vi "Lab Panel V4.85.vi"() -> ()   [LabVIEW 2013] (continued)
                            n1529 = local write "run lab03-2"(w2748) -> ()
                          }
                          frame #1 {
                            n1530 = TDMS Close(11:w2752) -> (0:w2753:errorcluster)  [unwired: 1 in, 1 out]
                            n1531 = local write "data file error"(w2753) -> ()
                          }
                          frame #2 {
                            n1532 = stacked-sequence {
                              tunnel: "LAB03-2" -> [w2761 w2762]
                              tunnel: w2758 -> [_ w2767]
                              tunnel: w2757 -> [_ w2766]
                              tunnel: w2756 -> [_ w2765]
                              tunnel: w2755 -> [_ w2764]
                              tunnel: w2754 -> [_ w2763]
                              frame #0 {
                                n1533 = call "sub vi - defrag tdms v1.vi"("panel id"=w2761) -> ("error out"=w2760:errorcluster)  [unwired: 10 in]
                                n1534 = local write "data file error"(w2760) -> ()
                              }
                              frame #1 {
                                n1535 = Bundle("STATUS"=w2767, "OUT SERVER ADDRESS"=w2766, "FROM ACCOUNT"=w2765, "Test File To"=w2764, "Mail Test Fail"=w2763) -> (w2769:T23)  [unwired: 1 in]
                                n1536 = call "Save data file to network drive v3.vi"("Input Cluster"=w2769, "panel id"=w2762) -> ("network file save error"=w2768:errorcluster)  [unwired: 8 in, 1 out]
                                n1537 = local write "data file error"(w2768) -> ()
                              }
                            }
                          }
                        }
                      }
                    }
                  }
                }
              }
              frame #6 {
                # "LAB04-1"
                n1538 = local read "run lab04-1"() -> (w2774:bool)
                n1539 = case shown="True" w2774 {
                  tunnel: w2773 -> [_ w2778]
                  tunnel: w2772 -> [_ w2777]
                  tunnel: w2771 -> [_ w2776]
                  tunnel: w2770 -> [_ w2775]
                  frame False {
                  }
                  frame True {
                    n1540 = local read "DISP LAB04-1"() -> (w2786:T4)
                    n1541 = Unbundle(w2786) -> ("CYCLE"=w2782:dbl, "STATUS"=w2779:string)  [unwired: 1 out]
                    n1542 = local read "TDMS LAB04-1"() -> (w2785:refnum<k34>)
                    n1543 = Not Equal?(x=w2779, y="RUN") -> (x != y?=w2781:bool)
                    n1544 = Greater?(x=w2782, y=2.0) -> (0:w2783:bool)
                    n1545 = And(x=w2783, y=w2781) -> (x .and. y?=w2780:bool)
                    n1546 = case shown="True" w2780 {
                      tunnel: w2786 -> [_ w2794]
                      tunnel: w2785 -> [_ w2793]
                      tunnel: w2779 -> [_ w2792]
                      tunnel: w2778 -> [_ w2791]
                      tunnel: w2777 -> [_ w2790]
                      tunnel: w2776 -> [_ w2789]
                      tunnel: w2775 -> [_ w2788]
                      frame False {
                      }
                      frame True {
                        n1547 = stacked-sequence {
                          tunnel: w2794 -> [w2797 _ _]
                          tunnel: w2793 -> [_ w2799 _]
                          tunnel: w2792 -> [_ _ w2805]
                          tunnel: w2791 -> [_ _ w2804]
                          tunnel: w2790 -> [_ _ w2803]
                          tunnel: w2789 -> [_ _ w2802]
                          tunnel: w2788 -> [_ _ w2801]
                          frame #0 {
                            w2795 = FALSE
                            n1548 = local write "mail control"("END") -> ()
                            n1549 = Bundle(cluster=w2797) -> (w2798:T4)  [unwired: 3 in]
                            n1550 = local write "RUN LAB04-1"(w2795) -> ()
                            n1551 = local write "O/I  LAB04-1"(w2795) -> ()
                            n1552 = local write "run lab04-1"(w2795) -> ()
                            n1553 = local write "DISP LAB04-1"(w2798) -> ()
                          }
                          frame #1 {
                            n1554 = TDMS Close(11:w2799) -> (0:w2800:errorcluster)  [unwired: 1 in, 1 out]
                            n1555 = local write "data file error"(w2800) -> ()
                          }
                          frame #2 {
                            n1556 = stacked-sequence {
                              tunnel: "LAB04-1" -> [w2808 w2809]
                              tunnel: w2805 -> [_ w2814]
                              tunnel: w2804 -> [_ w2813]
                              tunnel: w2803 -> [_ w2812]
                              tunnel: w2802 -> [_ w2811]
                              tunnel: w2801 -> [_ w2810]
                              frame #0 {
                                n1557 = call "sub vi - defrag tdms v1.vi"("panel id"=w2808) -> ("error out"=w2807:errorcluster)  [unwired: 10 in]
                                n1558 = local write "data file error"(w2807) -> ()
                              }
                              frame #1 {
                                n1559 = Bundle("STATUS"=w2814, "OUT SERVER ADDRESS"=w2813, "FROM ACCOUNT"=w2812, "Test File To"=w2811, "Mail Test Fail"=w2810) -> (w2816:T23)  [unwired: 1 in]
                                n1560 = call "Save data file to network drive v3.vi"("Input Cluster"=w2816, "panel id"=w2809) -> ("network file save error"=w2815:errorcluster)  [unwired: 8 in, 1 out]
                                n1561 = local write "data file error"(w2815) -> ()
                              }
                            }
                          }
                        }
                      }
                    }
                  }
                }
              }
              frame #7 {
                # "LAB04-2"
                n1562 = local read "run lab04-2"() -> (w2821:bool)
                n1563 = case shown="True" w2821 {
                  tunnel: w2820 -> [_ w2825]
                  tunnel: w2819 -> [_ w2824]
                  tunnel: w2818 -> [_ w2823]
                  tunnel: w2817 -> [_ w2822]
                  frame False {
                  }
                  frame True {
                    n1564 = local read "DISP LAB04-2"() -> (w2833:T4)
                    n1565 = Unbundle(w2833) -> ("CYCLE"=w2829:dbl, "STATUS"=w2826:string)  [unwired: 1 out]
                    n1566 = Not Equal?(x=w2826, y="RUN") -> (x != y?=w2828:bool)
                    n1567 = local read "TDMS LAB04-2"() -> (w2832:refnum<k34>)
                    n1568 = Greater?(x=w2829, y=2.0) -> (0:w2830:bool)
                    n1569 = And(x=w2830, y=w2828) -> (x .and. y?=w2827:bool)
                    n1570 = case shown="True" w2827 {
                      tunnel: w2833 -> [_ w2841]
                      tunnel: w2832 -> [_ w2840]
                      tunnel: w2826 -> [_ w2839]
                      tunnel: w2825 -> [_ w2838]
                      tunnel: w2824 -> [_ w2837]
                      tunnel: w2823 -> [_ w2836]
                      tunnel: w2822 -> [_ w2835]
                      frame False {
                      }
                      frame True {
                        n1571 = stacked-sequence {
                          tunnel: w2841 -> [w2844 _ _]
                          tunnel: w2840 -> [_ w2846 _]
                          tunnel: w2839 -> [_ _ w2852]
                          tunnel: w2838 -> [_ _ w2851]
                          tunnel: w2837 -> [_ _ w2850]
                          tunnel: w2836 -> [_ _ w2849]
                          tunnel: w2835 -> [_ _ w2848]
                          frame #0 {
                            w2842 = FALSE
                            n1572 = local write "mail control"("END") -> ()
                            n1573 = Bundle(cluster=w2844) -> (w2845:T4)  [unwired: 3 in]
                            n1574 = local write "O/I  LAB04-2"(w2842) -> ()
                            n1575 = local write "RUN LAB04-2"(w2842) -> ()
                            n1576 = local write "run lab04-2"(w2842) -> ()
                            n1577 = local write "DISP LAB04-2"(w2845) -> ()
                          }
                          frame #1 {
                            n1578 = TDMS Close(11:w2846) -> (0:w2847:errorcluster)  [unwired: 1 in, 1 out]
                            n1579 = local write "data file error"(w2847) -> ()
                          }
                          frame #2 {
                            n1580 = stacked-sequence {
                              tunnel: "LAB04-2" -> [w2855 w2856]
                              tunnel: w2852 -> [_ w2861]
                              tunnel: w2851 -> [_ w2860]
                              tunnel: w2850 -> [_ w2859]
                              tunnel: w2849 -> [_ w2858]
                              tunnel: w2848 -> [_ w2857]
                              frame #0 {
                                n1581 = call "sub vi - defrag tdms v1.vi"("panel id"=w2855) -> ("error out"=w2854:errorcluster)  [unwired: 10 in]
                                n1582 = local write "data file error"(w2854) -> ()
                              }
                              frame #1 {
                                n1583 = Bundle("STATUS"=w2861, "OUT SERVER ADDRESS"=w2860, "FROM ACCOUNT"=w2859, "Test File To"=w2858, "Mail Test Fail"=w2857) -> (w2863:T23)  [unwired: 1 in]
                                n1584 = call "Save data file to network drive v3.vi"("Input Cluster"=w2863, "panel id"=w2856) -> ("network file save error"=w2862:errorcluster)  [unwired: 8 in, 1 out]
                                n1585 = local write "data file error"(w2862) -> ()
                              }
                            }
                          }
                        }
                      }
                    }
                  }
                }
              }
              frame #8 {
                # "LAB05-1"
                n1586 = local read "run lab05-1"() -> (w2868:bool)
                n1587 = case shown="True" w2868 {
                  tunnel: w2867 -> [_ w2872]
                  tunnel: w2866 -> [_ w2871]
                  tunnel: w2865 -> [_ w2870]
                  tunnel: w2864 -> [_ w2869]
                  frame False {
                  }
                  frame True {
                    n1588 = local read "DISP LAB05-1"() -> (w2880:T4)
                    n1589 = Unbundle(w2880) -> ("CYCLE"=w2876:dbl, "STATUS"=w2873:string)  [unwired: 1 out]
                    n1590 = Not Equal?(x=w2873, y="RUN") -> (x != y?=w2875:bool)
                    n1591 = local read "TDMS LAB05-1"() -> (w2879:refnum<k34>)
                    n1592 = Greater?(x=w2876, y=2.0) -> (0:w2877:bool)
                    n1593 = And(x=w2877, y=w2875) -> (x .and. y?=w2874:bool)
                    n1594 = case shown="True" w2874 {
                      tunnel: w2880 -> [_ w2888]
                      tunnel: w2879 -> [_ w2887]
                      tunnel: w2873 -> [_ w2886]
                      tunnel: w2872 -> [_ w2885]
                      tunnel: w2871 -> [_ w2884]
                      tunnel: w2870 -> [_ w2883]
                      tunnel: w2869 -> [_ w2882]
                      frame False {
                      }
                      frame True {
                        n1595 = stacked-sequence {
                          tunnel: w2888 -> [w2891 _ _]
                          tunnel: w2887 -> [_ w2893 _]
                          tunnel: w2886 -> [_ _ w2899]
                          tunnel: w2885 -> [_ _ w2898]
                          tunnel: w2884 -> [_ _ w2897]
                          tunnel: w2883 -> [_ _ w2896]
                          tunnel: w2882 -> [_ _ w2895]
                          frame #0 {
                            w2889 = FALSE
                            n1596 = local write "mail control"("END") -> ()
                            n1597 = Bundle(cluster=w2891) -> (w2892:T4)  [unwired: 3 in]
                            n1598 = local write "O/I  LAB05-1"(w2889) -> ()
                            n1599 = local write "RUN LAB05-1"(w2889) -> ()
                            n1600 = local write "run lab05-1"(w2889) -> ()
                            n1601 = local write "DISP LAB05-1"(w2892) -> ()
                          }
                          frame #1 {
                            n1602 = TDMS Close(11:w2893) -> (0:w2894:errorcluster)  [unwired: 1 in, 1 out]
                            n1603 = local write "data file error"(w2894) -> ()
                          }
                          frame #2 {
                            n1604 = stacked-sequence {
                              tunnel: "LAB05-1" -> [w2902 w2908]
                              tunnel: w2899 -> [_ w2907]
                              tunnel: w2898 -> [_ w2906]
                              tunnel: w2897 -> [_ w2905]
                              tunnel: w2896 -> [_ w2904]
                              tunnel: w2895 -> [_ w2903]
                              frame #0 {
                                n1605 = call "sub vi - defrag tdms v1.vi"("panel id"=w2902) -> ("error out"=w2901:errorcluster)  [unwired: 10 in]
                                n1606 = local write "data file error"(w2901) -> ()
                              }
                              frame #1 {
                                n1607 = Bundle("STATUS"=w2907, "OUT SERVER ADDRESS"=w2906, "FROM ACCOUNT"=w2905, "Test File To"=w2904, "Mail Test Fail"=w2903) -> (w2910:T23)  [unwired: 1 in]
                                n1608 = call "Save data file to network drive v3.vi"("Input Cluster"=w2910, "panel id"=w2908) -> ("network file save error"=w2909:errorcluster)  [unwired: 8 in, 1 out]
                                n1609 = local write "data file error"(w2909) -> ()
                              }
                            }
                          }
                        }
                      }
                    }
                  }
                }
              }
              frame #9 {
                # "LAB05-2"
                n1610 = local read "run lab05-2"() -> (w2915:bool)
                n1611 = case shown="True" w2915 {
                  tunnel: w2914 -> [_ w2919]
                  tunnel: w2913 -> [_ w2918]
                  tunnel: w2912 -> [_ w2917]
                  tunnel: w2911 -> [_ w2916]
                  frame False {
                  }
                  frame True {
                    n1612 = local read "DISP LAB05-2"() -> (w2927:T4)
                    n1613 = Unbundle(w2927) -> ("CYCLE"=w2923:dbl, "STATUS"=w2920:string)  [unwired: 1 out]
                    n1614 = Not Equal?(x=w2920, y="RUN") -> (x != y?=w2922:bool)
                    n1615 = local read "TDMS LAB05-2"() -> (w2926:refnum<k34>)
                    n1616 = Greater?(x=w2923, y=2.0) -> (0:w2924:bool)
                    n1617 = And(x=w2924, y=w2922) -> (x .and. y?=w2921:bool)
                    n1618 = case shown="True" w2921 {
                      tunnel: w2927 -> [_ w2935]
                      tunnel: w2926 -> [_ w2934]
                      tunnel: w2920 -> [_ w2933]
                      tunnel: w2919 -> [_ w2932]
                      tunnel: w2918 -> [_ w2931]
                      tunnel: w2917 -> [_ w2930]
                      tunnel: w2916 -> [_ w2929]
                      frame False {
                      }
                      frame True {
                        n1619 = stacked-sequence {
                          tunnel: w2935 -> [w2938 _ _]
                          tunnel: w2934 -> [_ w2940 _]
                          tunnel: w2933 -> [_ _ w2946]
                          tunnel: w2932 -> [_ _ w2945]
                          tunnel: w2931 -> [_ _ w2944]
                          tunnel: w2930 -> [_ _ w2943]
                          tunnel: w2929 -> [_ _ w2942]
                          frame #0 {
                            w2936 = FALSE
                            n1620 = local write "mail control"("END") -> ()
                            n1621 = Bundle(cluster=w2938) -> (w2939:T4)  [unwired: 3 in]
                            n1622 = local write "RUN LAB05-2"(w2936) -> ()
                            n1623 = local write "O/I  LAB05-2"(w2936) -> ()
                            n1624 = local write "run lab05-2"(w2936) -> ()
                            n1625 = local write "DISP LAB05-2"(w2939) -> ()
                          }
                          frame #1 {
                            n1626 = TDMS Close(11:w2940) -> (0:w2941:errorcluster)  [unwired: 1 in, 1 out]
                            n1627 = local write "data file error"(w2941) -> ()
                          }
                          frame #2 {
                            n1628 = stacked-sequence {
                              tunnel: "LAB05-2" -> [w2949 w2955]
                              tunnel: w2946 -> [_ w2954]
                              tunnel: w2945 -> [_ w2953]
                              tunnel: w2944 -> [_ w2952]
                              tunnel: w2943 -> [_ w2951]
                              tunnel: w2942 -> [_ w2950]
                              frame #0 {
                                n1629 = call "sub vi - defrag tdms v1.vi"("panel id"=w2949) -> ("error out"=w2948:errorcluster)  [unwired: 10 in]
                                n1630 = local write "data file error"(w2948) -> ()
                              }
                              frame #1 {
                                n1631 = Bundle("STATUS"=w2954, "OUT SERVER ADDRESS"=w2953, "FROM ACCOUNT"=w2952, "Test File To"=w2951, "Mail Test Fail"=w2950) -> (w2957:T23)  [unwired: 1 in]
                                n1632 = call "Save data file to network drive v3.vi"("Input Cluster"=w2957, "panel id"=w2955) -> ("network file save error"=w2956:errorcluster)  [unwired: 8 in, 1 out]
                                n1633 = local write "data file error"(w2956) -> ()
                              }
                            }
                          }
                        }
                      }
                    }
                  }
                }
              }
            }
            n1634 = local read "Network Directory"() -> (w2471:path)
            n1635 = global write "Global 1.vi" "Network Drive"(w2471) -> ()
          }
          frame #7 {
            # "disable functions"
            n1636 = stacked-sequence {
              tunnel: w2967 -> [w2981 _ w3038]
              tunnel: w2966 -> [w2976 _ w3037]
              tunnel: w2965 -> [w2975 _ w3036]
              tunnel: w2964 -> [w2973 _ w3035]
              tunnel: w2963 -> [w2974 _ w3034]
              tunnel: w2962 -> [_ w2998 w3033]
              tunnel: w2961 -> [_ w2999 w3032]
              tunnel: w2960 -> [_ w3000 w3031]
              tunnel: w2959 -> [_ w3001 w3030]
              tunnel: w2958 -> [_ w3002 w3029]
              frame #0 {
                n1637 = Select(t=2, s=w2973, f=0) -> (s? t:f=w2969:i32)
                n1638 = Select(t=2, s=w2975, f=0) -> (s? t:f=w2970:i32)
                n1639 = Select(t=2, s=w2974, f=0) -> (s? t:f=w2968:i32)
                n1640 = Select(t=2, s=w2981, f=0) -> (s? t:f=w2972:i32)
                n1641 = Select(t=2, s=w2976, f=0) -> (s? t:f=w2971:i32)
                n1642 = property on="SELECT LAB02-2" class="RadioBtnsControl (strict)"("DisabledEnum"=w2969) -> ()  [unwired: 2 in, 2 out]
                n1643 = property on="SELECT LAB02-1" class="RadioBtnsControl (strict)"("DisabledEnum"=w2970) -> ()  [unwired: 2 in, 2 out]
                n1644 = property on="SELECT LAB03-1" class="RadioBtnsControl (strict)"("DisabledEnum"=w2968) -> ()  [unwired: 2 in, 2 out]
                n1645 = property on="SELECT LAB01-1" class="RadioBtnsControl (strict)"("DisabledEnum"=w2972) -> ()  [unwired: 2 in, 2 out]
                n1646 = property on="SELECT LAB01-2" class="RadioBtnsControl (strict)"("DisabledEnum"=w2971) -> ()  [unwired: 2 in, 2 out]
                n1647 = Not(x=w2981) -> (.not. x?=w2982:bool)
                n1648 = property on="RESULT LAB01-1" class="Bool (strict)"("Visible"=w2982) -> ()  [unwired: 2 in, 2 out]
                n1649 = Not(x=w2976) -> (.not. x?=w2980:bool)
                n1650 = Not(x=w2975) -> (.not. x?=w2979:bool)
                n1651 = Not(x=w2973) -> (.not. x?=w2978:bool)
                n1652 = property on="RESULT LAB01-2" class="Bool (strict)"("Visible"=w2980) -> ()  [unwired: 2 in, 2 out]
                n1653 = Not(x=w2974) -> (.not. x?=w2977:bool)
                n1654 = property on="RESULT LAB02-1" class="Bool (strict)"("Visible"=w2979) -> ()  [unwired: 2 in, 2 out]
                n1655 = property on="RESULT LAB02-2" class="Bool (strict)"("Visible"=w2978) -> ()  [unwired: 2 in, 2 out]
                n1656 = property on="RESULT LAB03-1" class="Bool (strict)"("Visible"=w2977) -> ()  [unwired: 2 in, 2 out]
                n1657 = property on="SET LAB01-1" class="Clust (strict)"("DisabledEnum"=w2972) -> ()  [unwired: 2 in, 2 out]
                n1658 = property on="SET LAB01-2" class="Clust (strict)"("DisabledEnum"=w2971) -> ()  [unwired: 2 in, 2 out]
                n1659 = property on="SET LAB02-1" class="Clust (strict)"("DisabledEnum"=w2970) -> ()  [unwired: 2 in, 2 out]
                n1660 = property on="SET LAB02-2" class="Clust (strict)"("DisabledEnum"=w2969) -> ()  [unwired: 2 in, 2 out]
                n1661 = property on="SET LAB03-1" class="Clust (strict)"("DisabledEnum"=w2968) -> ()  [unwired: 2 in, 2 out]
                n1662 = property on="O/I  LAB01-1" class="Bool (strict)"("DisabledEnum"=w2972) -> ()  [unwired: 2 in, 2 out]
                n1663 = property on="O/I  LAB01-2" class="Bool (strict)"("DisabledEnum"=w2971) -> ()  [unwired: 2 in, 2 out]
                n1664 = property on="O/I  LAB02-1" class="Bool (strict)"("DisabledEnum"=w2970) -> ()  [unwired: 2 in, 2 out]
                n1665 = property on="O/I  LAB02-2" class="Bool (strict)"("DisabledEnum"=w2969) -> ()  [unwired: 2 in, 2 out]
                n1666 = property on="O/I  LAB03-1" class="Bool (strict)"("DisabledEnum"=w2968) -> ()  [unwired: 2 in, 2 out]
              }
              frame #1 {
                n1667 = Select(t=2, s=w3002, f=0) -> (s? t:f=w2993:i32)
                n1668 = Select(t=2, s=w3001, f=0) -> (s? t:f=w2994:i32)
                n1669 = Select(t=2, s=w2998, f=0) -> (s? t:f=w2997:i32)
                n1670 = Select(t=2, s=w2999, f=0) -> (s? t:f=w2996:i32)
                n1671 = Select(t=2, s=w3000, f=0) -> (s? t:f=w2995:i32)
                n1672 = property on="SELECT LAB05-2" class="RadioBtnsControl (strict)"("DisabledEnum"=w2993) -> ()  [unwired: 2 in, 2 out]
                n1673 = property on="SELECT LAB05-1" class="RadioBtnsControl (strict)"("DisabledEnum"=w2994) -> ()  [unwired: 2 in, 2 out]
                n1674 = property on="SELECT LAB03-2" class="RadioBtnsControl (strict)"("DisabledEnum"=w2997) -> ()  [unwired: 2 in, 2 out]
                n1675 = property on="SELECT LAB04-1" class="RadioBtnsControl (strict)"("DisabledEnum"=w2996) -> ()  [unwired: 2 in, 2 out]
                n1676 = property on="SELECT LAB04-2" class="RadioBtnsControl (strict)"("DisabledEnum"=w2995) -> ()  [unwired: 2 in, 2 out]
                n1677 = property on="SET LAB05-2" class="Clust (strict)"("DisabledEnum"=w2993) -> ()  [unwired: 2 in, 2 out]
                n1678 = property on="SET LAB05-1" class="Clust (strict)"("DisabledEnum"=w2994) -> ()  [unwired: 2 in, 2 out]
                n1679 = property on="SET LAB03-2" class="Clust (strict)"("DisabledEnum"=w2997) -> ()  [unwired: 2 in, 2 out]
                n1680 = property on="SET LAB04-1" class="Clust (strict)"("DisabledEnum"=w2996) -> ()  [unwired: 2 in, 2 out]
                n1681 = property on="SET LAB04-2" class="Clust (strict)"("DisabledEnum"=w2995) -> ()  [unwired: 2 in, 2 out]
                n1682 = property on="O/I  LAB05-2" class="Bool (strict)"("DisabledEnum"=w2993) -> ()  [unwired: 2 in, 2 out]
                n1683 = property on="O/I  LAB05-1" class="Bool (strict)"("DisabledEnum"=w2994) -> ()  [unwired: 2 in, 2 out]
                n1684 = property on="O/I  LAB04-1" class="Bool (strict)"("DisabledEnum"=w2996) -> ()  [unwired: 2 in, 2 out]
                n1685 = property on="O/I  LAB04-2" class="Bool (strict)"("DisabledEnum"=w2995) -> ()  [unwired: 2 in, 2 out]
                n1686 = property on="O/I  LAB03-2" class="Bool (strict)"("DisabledEnum"=w2997) -> ()  [unwired: 2 in, 2 out]
                n1687 = Not(x=w3002) -> (.not. x?=w3003:bool)
                n1688 = Not(x=w3001) -> (.not. x?=w3004:bool)
                n1689 = Not(x=w3000) -> (.not. x?=w3005:bool)
                n1690 = property on="RESULT LAB05-2" class="Bool (strict)"("Visible"=w3003) -> ()  [unwired: 2 in, 2 out]
                n1691 = property on="RESULT LAB05-1" class="Bool (strict)"("Visible"=w3004) -> ()  [unwired: 2 in, 2 out]
                n1692 = Not(x=w2999) -> (.not. x?=w3006:bool)
                n1693 = property on="RESULT LAB04-2" class="Bool (strict)"("Visible"=w3005) -> ()  [unwired: 2 in, 2 out]
                n1694 = Not(x=w2998) -> (.not. x?=w3007:bool)
                n1695 = property on="RESULT LAB04-1" class="Bool (strict)"("Visible"=w3006) -> ()  [unwired: 2 in, 2 out]
                n1696 = property on="RESULT LAB03-2" class="Bool (strict)"("Visible"=w3007) -> ()  [unwired: 2 in, 2 out]
              }
              frame #2 {
                # "disable calibrate if any test running"
                n1697 = Or(x=w3030, y=w3029) -> (x .or. y?=w3023:bool)
                n1698 = Or(x=w3032, y=w3031) -> (x .or. y?=w3025:bool)
                n1699 = Or(x=w3036, y=w3035) -> (x .or. y?=w3027:bool)
                n1700 = Or(x=w3034, y=w3033) -> (x .or. y?=w3026:bool)
                n1701 = Or(x=w3038, y=w3037) -> (x .or. y?=w3028:bool)
                n1702 = Or(x=w3026, y=w3025) -> (x .or. y?=w3024:bool)
                n1703 = Or(x=w3028, y=w3027) -> (x .or. y?=w3022:bool)
                n1704 = Or(x=w3024, y=w3023) -> (x .or. y?=w3021:bool)
                n1705 = Or(x=w3022, y=w3021) -> (x .or. y?=w3020:bool)
                n1706 = case shown="False" w3020 {
                  tunnel: [0 2] -> w3019
                  frame False {
                  }
                  frame True {
                  }
                }
                n1707 = property on="JIG TEST" class="Clust (strict)"("DisabledEnum"=w3019) -> ()  [unwired: 2 in, 2 out]
                n1708 = property on="Network Directory" class="Path"("DisabledEnum"=w3019) -> ()  [unwired: 2 in, 2 out]
                n1709 = property on="MAIL SETTINGS" class="Clust (strict)"("DisabledEnum"=w3019) -> ()  [unwired: 2 in, 2 out]
                n1710 = property on="SET (cal)" class="Bool (strict)"("DisabledEnum"=w3019) -> ()  [unwired: 2 in, 2 out]
                n1711 = property on="ADMIN" class="Bool (strict)"("DisabledEnum"=0) -> ()  [unwired: 2 in, 2 out]
              }
            }
          }
          frame #8 {
            # "drive jigs"
            n1712 = stacked-sequence {
              frame #0 {
                # "jig on"
                n1713 = local read "jig cycle"() -> (w3046:dbl)
                n1714 = property on="JIG TEST" class="Clust (strict)"() -> ("DisabledEnum"=w3043:T14)  [unwired: 2 in, 2 out]
                n1715 = Equal?(x=w3043, y=2) -> (x = y?=w3042:bool)
                n1716 = Equal?(x=w3046, y=0) -> (x = y?=w3044:bool)
                n1717 = And(x=w3044, y=w3042) -> (x .and. y?=w3041:bool)
                n1718 = case shown="True" w3041 {
                  frame False {
                  }
                  frame True {
                    n1719 = local read "run lab01-1"() -> (w3057:bool)
                    n1720 = local read "run lab01-2"() -> (w3056:bool)
                    n1721 = local read "run lab02-1"() -> (w3055:bool)
                    n1722 = local read "run lab02-2"() -> (w3054:bool)
                    n1723 = local read "run lab03-1"() -> (w3053:bool)
                    n1724 = local read "run lab03-2"() -> (w3052:bool)
                    n1725 = local read "run lab04-1"() -> (w3051:bool)
                    n1726 = local read "run lab04-2"() -> (w3050:bool)
                    n1727 = local read "run lab05-1"() -> (w3049:bool)
                    n1728 = local read "run lab05-2"() -> (w3048:bool)
                    n1729 = local write "JIG LAB03-2"(w3052) -> ()
                    n1730 = local write "JIG LAB01-1"(w3057) -> ()
                    n1731 = local write "JIG LAB01-2"(w3056) -> ()
                    n1732 = local write "JIG LAB02-1"(w3055) -> ()
                    n1733 = local write "JIG LAB02-2"(w3054) -> ()
                    n1734 = local write "JIG LAB03-1"(w3053) -> ()
                    n1735 = local write "JIG LAB04-1"(w3051) -> ()
                    n1736 = local write "JIG LAB04-2"(w3050) -> ()
                    n1737 = local write "JIG LAB05-1"(w3049) -> ()
                    n1738 = local write "JIG LAB05-2"(w3048) -> ()
                  }
                }
              }
              frame #1 {
                # "jig off"
                n1739 = local read "jig cycle"() -> (w3064:dbl)
                n1740 = local read "on loops"() -> (w3063:dbl)
                n1741 = property on="JIG TEST" class="Clust (strict)"() -> ("DisabledEnum"=w3062:T14)  [unwired: 2 in, 2 out]
                n1742 = Equal?(x=w3062, y=2) -> (x = y?=w3060:bool)
                n1743 = Equal?(x=w3064, y=w3063) -> (x = y?=w3059:bool)
                n1744 = And(x=w3059, y=w3060) -> (x .and. y?=w3058:bool)
                n1745 = case shown="True" w3058 {
                  frame False {
                  }
                  frame True {
                    w3115 = FALSE
                    w3116 = TRUE
                    w3114 = 2
                    n1746 = local read "SELECT LAB05-2"() -> (w3105:T3)
                    n1747 = local read "SELECT LAB04-2"() -> (w3107:T3)
                    n1748 = local read "SELECT LAB04-1"() -> (w3108:T3)
                    n1749 = local read "SELECT LAB05-1"() -> (w3106:T3)
                    n1750 = local read "SELECT LAB03-2"() -> (w3109:T3)
                    n1751 = local read "SELECT LAB02-1"() -> (w3112:T3)
                    n1752 = local read "SELECT LAB03-1"() -> (w3110:T3)
                    n1753 = local read "SELECT LAB02-2"() -> (w3111:T3)
                    n1754 = local read "SELECT LAB01-2"() -> (w3113:T3)
                    n1755 = local read "run lab05-1"() -> (w3075:bool)
                    n1756 = local read "run lab05-2"() -> (w3074:bool)
                    n1757 = local read "SELECT LAB01-1"() -> (w3117:T3)
                    n1758 = local read "run lab04-2"() -> (w3076:bool)
                    n1759 = local read "run lab04-1"() -> (w3077:bool)
                    n1760 = local read "run lab01-1"() -> (w3093:bool)
                    n1761 = local read "run lab01-2"() -> (w3082:bool)
                    n1762 = local read "run lab03-2"() -> (w3078:bool)
                    n1763 = local read "run lab03-1"() -> (w3079:bool)
                    n1764 = local read "run lab02-1"() -> (w3081:bool)
                    n1765 = local read "run lab02-2"() -> (w3080:bool)
                    n1766 = Equal?(x=w3114, y=w3110) -> (x = y?=w3088:bool)
                    n1767 = Equal?(x=w3114, y=w3109) -> (x = y?=w3087:bool)
                    n1768 = Equal?(x=w3114, y=w3108) -> (x = y?=w3086:bool)
                    n1769 = Equal?(x=w3114, y=w3107) -> (x = y?=w3085:bool)
                    n1770 = Equal?(x=w3114, y=w3106) -> (x = y?=w3084:bool)
                    n1771 = Equal?(x=w3114, y=w3105) -> (x = y?=w3083:bool)
                    n1772 = Equal?(x=w3114, y=w3117) -> (x = y?=w3094:bool)
                    n1773 = Equal?(x=w3114, y=w3112) -> (x = y?=w3090:bool)
                    n1774 = Equal?(x=w3114, y=w3111) -> (x = y?=w3089:bool)
                    n1775 = Equal?(x=w3114, y=w3113) -> (x = y?=w3091:bool)
                    n1776 = And(x=w3085, y=w3076) -> (x .and. y?=w3067:bool)
                    n1777 = And(x=w3088, y=w3079) -> (x .and. y?=w3070:bool)
                    n1778 = And(x=w3086, y=w3077) -> (x .and. y?=w3068:bool)
                    n1779 = And(x=w3083, y=w3074) -> (x .and. y?=w3065:bool)
                    n1780 = And(x=w3089, y=w3080) -> (x .and. y?=w3071:bool)
                    n1781 = And(x=w3087, y=w3078) -> (x .and. y?=w3069:bool)
                    n1782 = And(x=w3084, y=w3075) -> (x .and. y?=w3066:bool)
                    n1783 = And(x=w3091, y=w3082) -> (x .and. y?=w3073:bool)
                    n1784 = And(x=w3094, y=w3093) -> (x .and. y?=w3092:bool)
                    n1785 = And(x=w3090, y=w3081) -> (x .and. y?=w3072:bool)
                    n1786 = Select(t=w3116, s=w3092, f=w3115) -> (s? t:f=w3095:bool)
                    n1787 = Select(t=w3116, s=w3073, f=w3115) -> (s? t:f=w3096:bool)
                    n1788 = Select(t=w3116, s=w3072, f=w3115) -> (s? t:f=w3097:bool)
                    n1789 = Select(t=w3116, s=w3071, f=w3115) -> (s? t:f=w3098:bool)
                    n1790 = Select(t=w3116, s=w3070, f=w3115) -> (s? t:f=w3099:bool)
                    n1791 = Select(t=w3116, s=w3069, f=w3115) -> (s? t:f=w3100:bool)
                    n1792 = Select(t=w3116, s=w3068, f=w3115) -> (s? t:f=w3101:bool)
                    n1793 = Select(t=w3116, s=w3067, f=w3115) -> (s? t:f=w3102:bool)
                    n1794 = Select(t=w3116, s=w3066, f=w3115) -> (s? t:f=w3103:bool)
                    n1795 = Select(t=w3116, s=w3065, f=w3115) -> (s? t:f=w3104:bool)
                    n1796 = local write "JIG LAB03-2"(w3100) -> ()
                    n1797 = local write "JIG LAB02-1"(w3097) -> ()
                    n1798 = local write "JIG LAB02-2"(w3098) -> ()
                    n1799 = local write "JIG LAB01-2"(w3096) -> ()
                    n1800 = local write "JIG LAB03-1"(w3099) -> ()
                    n1801 = local write "JIG LAB01-1"(w3095) -> ()
                    n1802 = local write "JIG LAB05-2"(w3104) -> ()
                    n1803 = local write "JIG LAB04-1"(w3101) -> ()
                    n1804 = local write "JIG LAB05-1"(w3103) -> ()
                    n1805 = local write "JIG LAB04-2"(w3102) -> ()
                  }
                }
              }
            }
          }
          frame #9 {
            # "enable  jig test output if no test busy"
            n1806 = property on="JIG TEST" class="Clust (strict)"() -> ("DisabledEnum"=w3120:T14)  [unwired: 2 in, 2 out]
            n1807 = Equal?(x=w3120, y=0) -> (x = y?=w3118:bool)
            n1808 = case shown="True" w3118 {
              frame False {
              }
              frame True {
                n1809 = local read "JIG TEST"() -> (w3131:T9)
                n1810 = Unbundle(w3131) -> ("LAB01-1"=w3130:bool, "LAB01-2"=w3129:bool, "LAB02-1"=w3128:bool, "LAB02-2"=w3127:bool, "LAB03-1"=w3126:bool, "LAB03-2"=w3125:bool, "LAB04-1"=w3124:bool, "LAB04-2"=w3123:bool, "LAB05-1"=w3122:bool, "LAB05-2"=w3121:bool)
                n1811 = local write "JIG LAB05-1"(w3122) -> ()
                n1812 = local write "JIG LAB05-2"(w3121) -> ()
                n1813 = local write "JIG LAB04-1"(w3124) -> ()
                n1814 = local write "JIG LAB04-2"(w3123) -> ()
                n1815 = local write "JIG LAB03-2"(w3125) -> ()
                n1816 = local write "JIG LAB01-1"(w3130) -> ()
                n1817 = local write "JIG LAB02-1"(w3128) -> ()
                n1818 = local write "JIG LAB03-1"(w3126) -> ()
                n1819 = local write "JIG LAB01-2"(w3129) -> ()
                n1820 = local write "JIG LAB02-2"(w3127) -> ()
              }
            }
          }
          frame #10 {
            # "drive digital output"
            n1821 = local read "O/I  LAB05-2"() -> (w3138:bool)
            n1822 = local read "O/I  LAB05-1"() -> (w3140:bool)
            n1823 = local read "JIG LAB05-2"() -> (w3137:bool)
            n1824 = local read "O/I  LAB04-2"() -> (w3142:bool)
            n1825 = local read "JIG LAB05-1"() -> (w3139:bool)
            n1826 = local read "JIG LAB04-2"() -> (w3141:bool)
            n1827 = local read "O/I  LAB03-1"() -> (w3147:bool)
            n1828 = local read "O/I  LAB04-1"() -> (w3143:bool)
            n1829 = local read "O/I  LAB02-1"() -> (w3151:bool)
            n1830 = local read "O/I  LAB02-2"() -> (w3149:bool)
            n1831 = local read "O/I  LAB03-2"() -> (w3145:bool)
            n1832 = local read "JIG LAB04-1"() -> (w3136:bool)
            n1833 = local read "JIG LAB03-2"() -> (w3144:bool)
            n1834 = local read "O/I  LAB01-2"() -> (w3153:bool)
            n1835 = local read "JIG LAB02-1"() -> (w3150:bool)
            n1836 = local read "JIG LAB02-2"() -> (w3148:bool)
            n1837 = local read "JIG LAB03-1"() -> (w3146:bool)
            n1838 = local read "O/I  LAB01-1"() -> (w3155:bool)
            n1839 = local read "JIG LAB01-2"() -> (w3152:bool)
            n1840 = local read "JIG LAB01-1"() -> (w3154:bool)
            n1841 = Build Array(w3142, w3141, w3140, w3139, w3138, w3137) -> (w3133:bool[])
            n1842 = Build Array(w3148, w3147, w3146, w3145, w3144, w3143, w3136) -> (w3134:bool[])
            n1843 = Build Array(w3155, w3154, w3153, w3152, w3151, w3150, w3149) -> (w3135:bool[])
            n1844 = local read "simulate"() -> (w3132:bool)
            n1845 = case shown="False" w3132 {
              tunnel: w3135 -> [w3158 _]
              tunnel: w3134 -> [w3157 _]
              tunnel: w3133 -> [w3156 _]
              frame False {
                n1846 = call "sub vi - Drive Relays All v6.vi"("Array #2"=w3156, "Array #1"=w3157, "Array #0"=w3158) -> ()  [unwired: 8 in, 1 out]
              }
              frame True {
              }
            }
          }
          frame #11 {
            # "get analog values"
            n1847 = local read "on loops"() -> (w3165:dbl)
            n1848 = local read "jig cycle"() -> (w3162:dbl)
            n1849 = Add(x=w3165, y=1) -> (x+y=w3163:dbl)
            n1850 = Equal?(x=w3162, y=1) -> (x = y?=w3160:bool)
            n1851 = Equal?(x=w3162, y=w3163) -> (x = y?=w3161:bool)
            n1852 = Or(x=w3160, y=w3161) -> (x .or. y?=w3159:bool)
            n1853 = case shown="True" w3159 {
              frame False {
              }
              frame True {
                n1854 = local read "simulate"() -> (w3169:bool)
                n1855 = case shown="False" w3169 {
                  tunnel: [w3185 errorcluster[] [] ("array ERROR")] -> w3177
                  tunnel: [w3184 0.3 ("Analog loop time")] -> w3176
                  tunnel: [w3183 dynamicdata[] [] ("array GRAPH")] -> w3175
                  tunnel: [w3182 w3187] -> w3174
                  tunnel: [w3181 w3187] -> w3173
                  tunnel: [w3180 w3187] -> w3172
                  tunnel: [w3179 w3187] -> w3171
                  tunnel: [w3178 w3187] -> w3170
                  frame False {
                    n1856 = call "sub vi - Read Analog All v8.vi"() -> ("Analog loop time"=w3184:dbl, "array GRAPH"=w3183:dynamicdata[], "LAB01"=w3182:T24, "LAB02"=w3181:T25, "LAB03"=w3180:T26, "LAB04"=w3179:T27, "array ERROR"=w3185:errorcluster[], "LAB05"=w3178:T28)  [unwired: 8 in]
                  }
                  frame True {
                    w3187 = T28 {"LAB05-1 (A)"=10.0, "LAB05-1 (V)"=220.0, "LAB05-1 (PF)"=0.5, "LAB05-2 (A)"=15.0, "LAB05-2 (V)"=225.0, "LAB05-2 (PF)"=0.6} ("LAB05")
                  }
                }
                n1857 = local read "simulate"() -> (w3168:bool)
                n1858 = stacked-sequence {
                  tunnel: w3177 -> [w3194 _ _ _ _ _]
                  tunnel: w3176 -> [w3193 _ _ _ _ _]
                  tunnel: w3175 -> [w3192 _ _ _ _ _]
                  tunnel: w3174 -> [_ w3241 _ _ _ _]
                  tunnel: w3173 -> [_ _ w3248 _ _ _]
                  tunnel: w3172 -> [_ _ _ w3277 _ _]
                  tunnel: w3171 -> [_ _ _ _ w3304 _]
                  tunnel: w3170 -> [_ _ _ _ _ w3333]
                  tunnel: w3168 -> [_ w3219 w3247 w3275 w3303 w3331]
                  tunnel: T12 {"1  (A) cal"=1.0, "1 (V) cal"=1.0, "1 (PF) cal"=1.0, "1 (TL) cal"=1.0, "1 (TN) cal"=1.0, "2 (A) cal"=1.0, "2 (V) cal"=1.0, "2 (PF) cal"=1.0, "2 (TL) cal"=1.0, "2 (TN) cal"=1.0} ("CAL LAB01") -> [_ w3218 w3246 w3274 w3302 w3330]
                  frame #0 {
                    n1859 = local write "AI"(TRUE) -> ()
                    n1860 = global write "Global 1.vi" "RATE(Hz)"("RATE (Hz)") -> ()
                    n1861 = global write "Global 1.vi" "SAMPLES"("SAMPLES") -> ()
                    n1862 = Index Array(array=w3192, index=6) -> (element=→"LAB04-1 (GRAPH)":dynamicdata)
                    n1863 = Index Array(array=w3192, index=7) -> (element=→"LAB04-2 (GRAPH)":dynamicdata)
                    n1864 = Index Array(array=w3192, index=9) -> (element=→"LAB05-2 (GRAPH)":dynamicdata)
                    n1865 = Index Array(array=w3192, index=8) -> (element=→"LAB05-1 (GRAPH)":dynamicdata)
                    n1866 = Index Array(array=w3192, index=5) -> (element=→"LAB03-2 (GRAPH)":dynamicdata)
                    n1867 = Index Array(array=w3192, index=0) -> (element=→"LAB01-1 (GRAPH)":dynamicdata)
                    n1868 = Index Array(array=w3192, index=1) -> (element=→"LAB01-2 (GRAPH)":dynamicdata)
                    n1869 = Index Array(array=w3192, index=2) -> (element=→"LAB02-1 (GRAPH)":dynamicdata)
                    n1870 = Index Array(array=w3192, index=3) -> (element=→"LAB02-2 (GRAPH)":dynamicdata)
                    n1871 = Index Array(array=w3192, index=4) -> (element=→"LAB03-1 (GRAPH)":dynamicdata)
                    "AI loop time" <- w3193
                    "Analog Error Array" <- w3194
                  }
                  frame #1 {
                    n1872 = Unbundle By Name(w3241) -> ("LAB05-1 (A)"=w3239:dbl, "LAB05-1 (V)"=w3238:dbl, "LAB05-1 (PF)"=w3237:dbl, "LAB05-2 (A)"=w3236:dbl, "LAB05-2 (V)"=w3235:dbl, "LAB05-2 (PF)"=w3234:dbl)
                    n1873 = case shown="False" w3219 {
                      tunnel: [w3242 w3243] -> w3240
                      tunnel: w3218 -> [_ w3243]
                      frame False {
                        n1874 = local read "CAL LAB01"() -> (w3242:T12)
                      }
                      frame True {
                      }
                    }
                    n1875 = Unbundle By Name(w3240) -> ("1  (A) cal"=w3233:dbl, "1 (V) cal"=w3232:dbl, "1 (PF) cal"=w3231:dbl, "2 (A) cal"=w3230:dbl, "2 (V) cal"=w3229:dbl, "2 (PF) cal"=w3228:dbl)  [unwired: 4 out]
                    n1876 = Multiply(x=w3239, y=w3233) -> (x*y=w3226:dbl)
                    n1877 = Multiply(x=w3238, y=w3232) -> (x*y=w3225:dbl)
                    n1878 = Multiply(x=w3237, y=w3231) -> (x*y=w3224:dbl)
                    n1879 = Multiply(x=w3236, y=w3230) -> (x*y=w3222:dbl)
                    n1880 = Multiply(x=w3235, y=w3229) -> (x*y=w3221:dbl)
                    n1881 = Multiply(x=w3234, y=w3228) -> (x*y=w3220:dbl)
                    n1882 = local read "SIG LAB01-1"() -> (w3227:T2)
                    n1883 = local read "SIG LAB01-2"() -> (w3223:T2)
                    n1884 = Bundle By Name(cluster=w3227, "AMPS"=w3226, "VOLTS"=w3225, "PF"=w3224) -> (w3217:T2)
                    n1885 = Bundle By Name(cluster=w3223, "AMPS"=w3222, "VOLTS"=w3221, "PF"=w3220) -> (w3216:T2)
                    n1886 = global write "Global display 1.vi" "SIG LAB01-2"(w3216) -> ()
                    n1887 = global write "Global display 1.vi" "SIG LAB01-1"(w3217) -> ()
                    n1888 = local write "SIG LAB01-2"(w3216) -> ()
                    n1889 = local write "SIG LAB01-1"(w3217) -> ()
                  }
                  frame #2 {
                    n1890 = Unbundle By Name(w3248) -> ("LAB05-1 (A)"=w3268:dbl, "LAB05-1 (V)"=w3267:dbl, "LAB05-1 (PF)"=w3266:dbl, "LAB05-2 (A)"=w3265:dbl, "LAB05-2 (V)"=w3264:dbl, "LAB05-2 (PF)"=w3263:dbl)
                    n1891 = case shown="True" w3247 {
                      tunnel: [w3270 w3271] -> w3269
                      tunnel: w3246 -> [_ w3271]
                      frame False {
                        n1892 = local read "CAL LAB02"() -> (w3270:T13)
                      }
                      frame True {
                      }
                    }
                    n1893 = Unbundle By Name(w3269) -> ("1  (A) cal"=w3262:dbl, "1 (V) cal"=w3261:dbl, "1 (PF) cal"=w3260:dbl, "2 (A) cal"=w3259:dbl, "2 (V) cal"=w3258:dbl, "2 (PF) cal"=w3257:dbl)  [unwired: 4 out]
                    n1894 = Multiply(x=w3268, y=w3262) -> (x*y=w3255:dbl)
                    n1895 = Multiply(x=w3267, y=w3261) -> (x*y=w3254:dbl)
                    n1896 = Multiply(x=w3266, y=w3260) -> (x*y=w3253:dbl)
                    n1897 = Multiply(x=w3265, y=w3259) -> (x*y=w3251:dbl)
                    n1898 = Multiply(x=w3264, y=w3258) -> (x*y=w3250:dbl)
                    n1899 = Multiply(x=w3263, y=w3257) -> (x*y=w3249:dbl)
                    n1900 = local read "SIG LAB02-1"() -> (w3256:T2)
                    n1901 = local read "SIG LAB02-2"() -> (w3252:T2)
                    n1902 = Bundle By Name(cluster=w3256, "AMPS"=w3255, "VOLTS"=w3254, "PF"=w3253) -> (w3245:T2)
                    n1903 = Bundle By Name(cluster=w3252, "AMPS"=w3251, "VOLTS"=w3250, "PF"=w3249) -> (w3244:T2)
                    n1904 = global write "Global display 1.vi" "SIG LAB02-1"(w3245) -> ()
                    n1905 = local write "SIG LAB02-2"(w3244) -> ()
                    n1906 = global write "Global display 1.vi" "SIG LAB02-2"(w3244) -> ()
                    n1907 = local write "SIG LAB02-1"(w3245) -> ()
                  }
                  frame #3 {
                    n1908 = Unbundle By Name(w3277) -> ("LAB05-1 (A)"=w3296:dbl, "LAB05-1 (V)"=w3295:dbl, "LAB05-1 (PF)"=w3294:dbl, "LAB05-2 (A)"=w3293:dbl, "LAB05-2 (V)"=w3292:dbl, "LAB05-2 (PF)"=w3291:dbl)
                    n1909 = case shown="True" w3275 {
                      tunnel: [w3298 w3299] -> w3297
                      tunnel: w3274 -> [_ w3299]
                      frame False {
                        n1910 = local read "CAL LAB03"() -> (w3298:T12)
                      }
                      frame True {
                      }
                    }
                    n1911 = Unbundle By Name(w3297) -> ("1  (A) cal"=w3290:dbl, "1 (V) cal"=w3289:dbl, "1 (PF) cal"=w3288:dbl, "2 (A) cal"=w3287:dbl, "2 (V) cal"=w3286:dbl, "2 (PF) cal"=w3285:dbl)  [unwired: 4 out]
                    n1912 = Multiply(x=w3296, y=w3290) -> (x*y=w3283:dbl)
                    n1913 = Multiply(x=w3295, y=w3289) -> (x*y=w3276:dbl)
                    n1914 = Multiply(x=w3294, y=w3288) -> (x*y=w3282:dbl)
                    n1915 = Multiply(x=w3293, y=w3287) -> (x*y=w3280:dbl)
                    n1916 = Multiply(x=w3292, y=w3286) -> (x*y=w3279:dbl)
                    n1917 = Multiply(x=w3291, y=w3285) -> (x*y=w3278:dbl)
                    n1918 = local read "SIG LAB03-1"() -> (w3284:T2)
                    n1919 = local read "SIG LAB03-2"() -> (w3281:T2)
                    n1920 = Bundle By Name(cluster=w3284, "AMPS"=w3283, "VOLTS"=w3276, "PF"=w3282) -> (w3273:T2)
                    n1921 = Bundle By Name(cluster=w3281, "AMPS"=w3280, "VOLTS"=w3279, "PF"=w3278) -> (w3272:T2)
                    n1922 = global write "Global display 1.vi" "SIG LAB03-1"(w3273) -> ()
                    n1923 = global write "Global display 1.vi" "SIG LAB03-2"(w3272) -> ()
                    n1924 = local write "SIG LAB03-2"(w3272) -> ()
                    n1925 = local write "SIG LAB03-1"(w3273) -> ()
                  }
                  frame #4 {
                    n1926 = Unbundle By Name(w3304) -> ("LAB05-1 (A)"=w3324:dbl, "LAB05-1 (V)"=w3323:dbl, "LAB05-1 (PF)"=w3322:dbl, "LAB05-2 (A)"=w3321:dbl, "LAB05-2 (V)"=w3320:dbl, "LAB05-2 (PF)"=w3319:dbl)
                    n1927 = case shown="False" w3303 {
                      tunnel: [w3326 w3327] -> w3325
                      tunnel: w3302 -> [_ w3327]
                      frame False {
                        n1928 = local read "CAL LAB04"() -> (w3326:T12)
                      }
                      frame True {
                      }
                    }
